vi "RCV Test_ks5080A.vi"(0 "Semiconductor Module Context":T2, 1 "Meas Type":T6, 2 "Test Information":T5={"Exp Name"="Cold Switching", "Lot"="0233A", "Wafer"="15", "Die Type"="L22", "Die X "="6", "Die Y"="8", "Exp"="1", "Die X_Y"="8"}, 3 "# of Cycles":string, 5 "Sweep Settings":T3={"Start"=0.0, "Stop"=1.0, "Step"=0.0}, 7 "Test_Pins":T4={"RF_Pins"=["RF1", "RF2"], "Contact_Meas_Pins"=["RF1"], "Contact_Source_Pins"=["RF1"], "Sweep_Bias_Pins"=[]}, 9 "error in (no error)":errorcluster, 12 "Averaging Count":i32=3, 13 "Plots FilePath":path=path "C:/Users/DalLab/Desktop/Test Data/Plots") -> (4 "ks5080A_Meaurements":T7, 15 "error out":errorcluster)   [LabVIEW 2013]
doc: "Initiates and fetches niVNA S11 measurements and converts it to a capacitance measurement."
uses:
  <vilib>/NI_TestStand_SemiconductorModule/NI_TestStand_Semiconductor_Module.lvlibp/PinMap/General/SemiconductorModuleContext.ctl
  Controls/Sweep Settings.ctl
  Controls/Test_Pins.ctl
  Controls/Test Information.ctl
  Controls/Meas Type.ctl
  Controls/ks5080A_Measurements.ctl
  <vilib>/NI_TestStand_SemiconductorModule/NI_TestStand_Semiconductor_Module.lvlibp
panel:
  in  "Tab Control":enum32{"Graphs", "Controls and Indicators"}(tab)
  out "Graph Cluster":T1
  out "Wafer":string
  out "Die Type":string
  out "Measurement":string
  out "Die X_Y":string
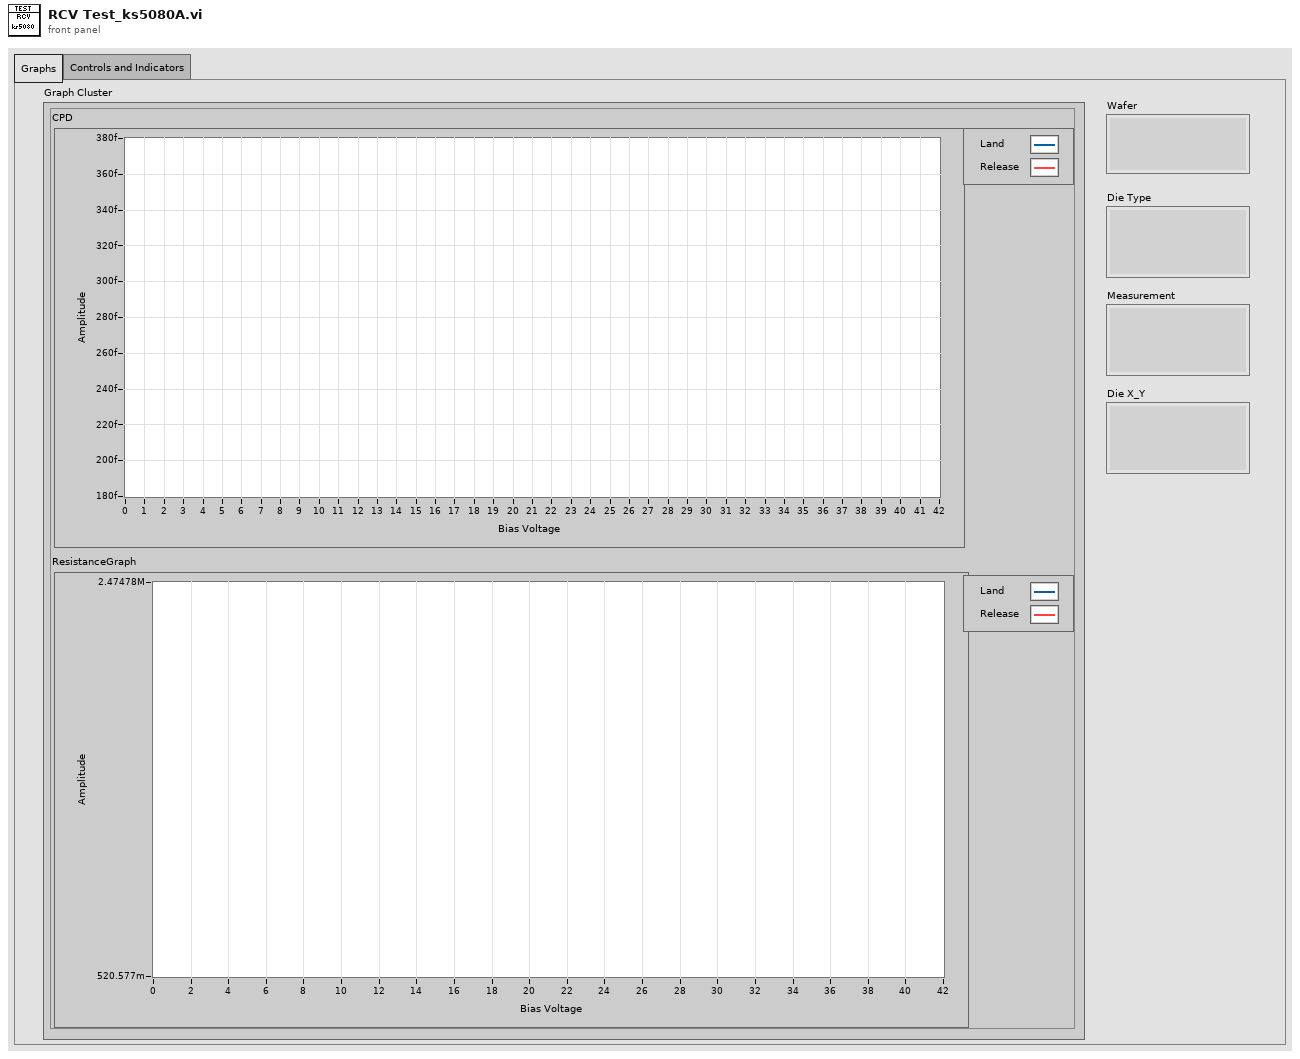
[diagram p1: front panel]
types:
  T1 = cluster{"ResistanceGraph":cluster{dbl[], dbl[]}[], "CPD":cluster{dbl[], dbl[]}[]}
  T2 = typedef "NI_TestStand_Semiconductor_Module.lvlibp/SemiconductorModuleContext.ctl" = refnum<k7>
  T3 = typedef "Sweep Settings.ctl" = cluster{"Start":dbl, "Stop":dbl, "Step":dbl}
  T4 = typedef "Test_Pins.ctl" = cluster{"RF_Pins":string[], "Contact_Meas_Pins":string[], "Contact_Source_Pins":string[], "Sweep_Bias_Pins":string[]}
  T5 = typedef "Test Information.ctl" = cluster{"Exp Name":string, "Lot":string, "Wafer":string, "Die Type":string, "Die X ":string, "Die Y":string, "Exp":string, "Die X_Y":string}
  T6 = typedef "Meas Type.ctl" = enum16{"Floor", "Roof", "Buckling", "Charge Transfer"}
  T7 = typedef "ks5080A_Measurements.ctl" = cluster{"Bias_Sweep_Setting":dbl[], "Bias_voltage measurements":dbl[], "Bias_current measurements":dbl[], "P1_Capacitance":dbl[], "P2_Capacitance":dbl[], "DMM_Measurement_V":dbl[], "Contact_Source Current measurements":dbl[], "Contact_Sink Current measurements":dbl[], "Calculated_Resistance":dbl[], "P3_Capacitance":dbl[], "Port 1_S_parm":string[], "Port 2_S_parm":string[], "Port 3_S_parm":string[]}
  T8 = typedef "ENA_Marker Measurements.ctl" = cluster{"Port 1 Capacitance":dbl[], "Port 2 Capacitance":dbl[], "Port 3 Capacitance":dbl[], "Port 1_S_parm":string[], "Port 2_S_parm":string[], "Port 3_S_parm":string[]}
  T9 = typedef "imagedata.ctl" = cluster{"image type":i32, "image depth":i32, "image":u8[], "mask":u8[], "colors":u32[], "Rectangle":cluster{"left":i16, "top":i16, "right":i16, "bottom":i16}}
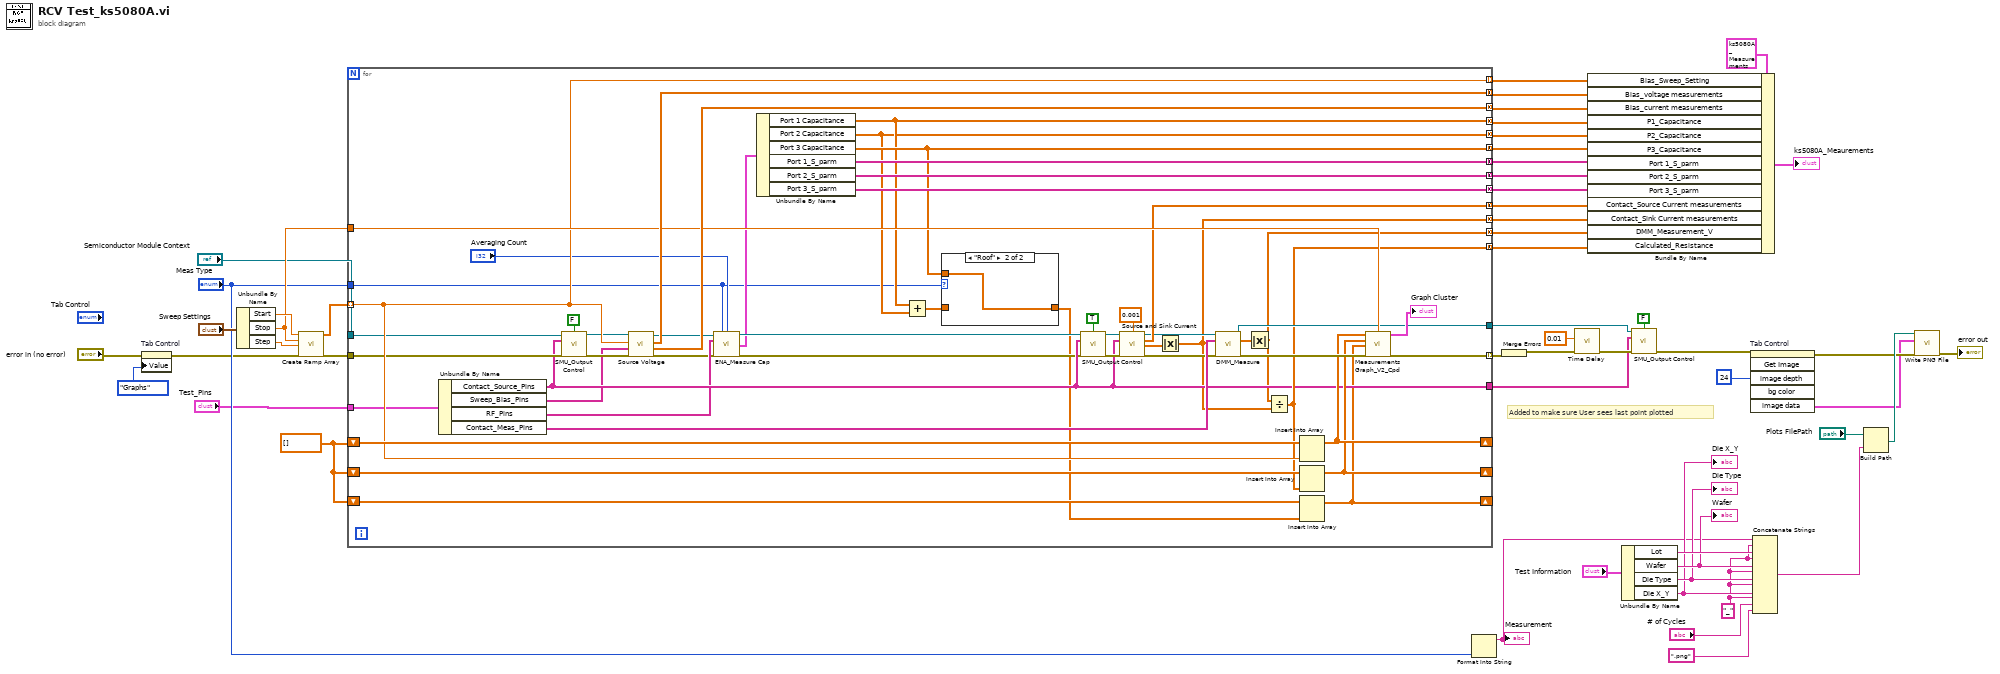
[diagram p0: block diagram]
diagram:
  w6 = "_"
  w46 = dbl[] []
  # "Added to make sure User sees last point plotted"
  n1 = property on="Tab Control" class="TabCtl (strict)"(error in="error in (no error)", "Value"=enum32{"Graphs", "Controls and Indicators"}."Graphs" ("Tab Control")) -> (error out=w7:errorcluster)  [unwired: 1 in, 1 out]
  n2 = Unbundle By Name("Sweep Settings") -> ("Start"=w49:dbl, "Stop"=w47:dbl, "Step"=w48:dbl)
  n3 = call "Create Ramp Array.vi"("Start"=w49, "Stop"=w47, "Step"=w48, "Error In"=w7) -> ("Ramp Pattern"=w52:dbl[], "Error Out"=w2:errorcluster)  [unwired: 10 in]
  n4 = for {
    tunnel: w52 -> [w91] mode=indexing
    tunnel: [w103] -> w38 mode=concatenating
    tunnel: [w102] -> w37 mode=concatenating
    tunnel: [w60] -> w34 mode=concatenating
    tunnel: [w100] -> w51 mode=indexing
    tunnel: w2 -> [w90]
    tunnel: w47 -> [w97]
    shift-right: [w96] -> _
    shift-left: w46 -> [w95]
    shift-right: [w94] -> _
    shift-left: w46 -> [w93]
    shift-right: [w76] -> _
    shift-left: w46 -> [w92]
    tunnel: [w91] -> w39 mode=indexing
    tunnel: [w84] -> w41
    tunnel: [w77] -> w40
    tunnel: [w83] -> w36 mode=concatenating
    tunnel: [w57] -> w35 mode=concatenating
    tunnel: [w82] -> w33 mode=concatenating
    tunnel: [w62] -> w21 mode=concatenating
    tunnel: [w61] -> w20 mode=concatenating
    tunnel: [w63] -> w19 mode=concatenating
    tunnel: [w66] -> w18 mode=concatenating
    tunnel: [w65] -> w17 mode=concatenating
    tunnel: [w64] -> w16 mode=concatenating
    tunnel: "Meas Type" -> [w56]
    tunnel: "Semiconductor Module Context" -> [w54]
    tunnel: "Test_Pins" -> [w53]
    n5 = Unbundle By Name(w53) -> ("Contact_Source_Pins"=w77:string[], "Sweep_Bias_Pins"=w75:string[], "RF_Pins"=w73:string[], "Contact_Meas_Pins"=w98:string[])
    n6 = call "SMU_Output Control.vi"("Semiconductor Module Context"=w54, "output enabled?"=FALSE, "Pins"=w77, "error in (no error)"=w90) -> ("Semiconductor Module Context Out"=w88:T2, "error out"=w89:errorcluster)  [unwired: 10 in]
    n7 = call "Source Voltage.vi"("error in (no error)"=w89, "Pins"=w75, "voltage level"=w91, "Semiconductor Module Context"=w88) -> ("error out"=w55:errorcluster, "current measurements"=w102:dbl[], "voltage measurements"=w103:dbl[], "Semiconductor Module Context Out"=w72:T2)  [unwired: 4 in]
    n8 = call "ENA_Measure Cap.vi"("Semiconductor Module Context"=w72, "Meas Type"=w56, "Averaging Count"="Averaging Count", "Pins"=w73, "error in (no error)"=w55) -> ("Semiconductor Module Context Out"=w71:T2, "Marker Measurements"=w67:T8, "error out"=w74:errorcluster)  [unwired: 8 in]
    n9 = Unbundle By Name(w67) -> ("Port 1 Capacitance"=w62:dbl[], "Port 2 Capacitance"=w61:dbl[], "Port 3 Capacitance"=w63:dbl[], "Port 1_S_parm"=w66:string[], "Port 2_S_parm"=w65:string[], "Port 3_S_parm"=w64:string[])
    n10 = Add(x=w62, y=w61) -> (x+y=w70:dbl[])
    n11 = case shown="\"Roof\"" w56 {
      tunnel: w70 -> [w104 _]
      tunnel: [w104 w105] -> w68
      tunnel: w63 -> [_ w105]
      frame "Floor", Default {
      }
      frame "Roof" {
      }
    }
    n12 = call "SMU_Output Control.vi"("Semiconductor Module Context"=w71, "output enabled?"=TRUE, "Pins"=w77, "error in (no error)"=w74) -> ("Semiconductor Module Context Out"=w78:T2, "error out"=w79:errorcluster)  [unwired: 10 in]
    n13 = call "Source and Sink Current.vi"("Semiconductor Module Context"=w78, "Current level"=0.001, "Pins"=w77, "error in (no error)"=w79) -> ("Semiconductor Module Context Out"=w80:T2, "Source Current measurements"=w83:dbl[], "Sink Current measurements"=w58:dbl[], "error out"=w81:errorcluster)  [unwired: 8 in]
    n14 = Absolute Value(x=w58) -> (abs(x)=w57:dbl[])
    n15 = call "DMM_Measure.vi"("Semiconductor Module Context"=w80, "Pins"=w98, "Error In"=w81) -> ("Semiconductor Module Context Out"=w84:T2, "Measurement"=w59:dbl[], "Error Out"=w101:errorcluster)  [unwired: 10 in]
    n16 = Absolute Value(x=w59) -> (abs(x)=w60:dbl[])
    n17 = Divide(x=w60, y=w57) -> (x/y=w82:dbl[])
    n18 = Insert Into Array(array=w95, new element=w91) -> (w96:dbl[])  [unwired: 1 in]
    n19 = Insert Into Array(array=w93, new element=w82) -> (w94:dbl[])  [unwired: 1 in]
    n20 = Insert Into Array(array=w92, new element=w68) -> (w76:dbl[])  [unwired: 1 in]
    n21 = call "Measurements Graph_V2_Cpd.vi"("Bias Voltage"=w96, "Stop_V"=w97, "Resitance"=w94, "Cpd"=w76, "Error In"=w101) -> ("Graph Cluster"=→"Graph Cluster":T1, "Error Out"=w100:errorcluster)  [unwired: 9 in]
  }
  n22 = Format Into String("Meas Type") -> (resulting string=w15:string)  [unwired: 3 in, 1 out]
  "Measurement" <- w15
  n23 = Merge Errors(w51) -> (w44:errorcluster)
  n24 = call "Time Delay"("error in (no error)"=w44, "Delay Time (s)"=0.01) -> ("error out"=w42:errorcluster)  [unwired: 9 in]
  n25 = Bundle By Name(cluster=T7 {"Bias_Sweep_Setting"=[], "Bias_voltage measurements"=[], "Bias_current measurements"=[], "P1_Capacitance"=[], "P2_Capacitance"=[], "DMM_Measurement_V"=[], "Contact_Source Current measurements"=[], "Contact_Sink Current measurements"=[], "Calculated_Resistance"=[], "P3_Capacitance"=[], "Port 1_S_parm"=[], "Port 2_S_parm"=[], "Port 3_S_parm"=[]} ("ks5080A_Meaurements 2"), "Bias_Sweep_Setting"=w39, "Bias_voltage measurements"=w38, "Bias_current measurements"=w37, "P1_Capacitance"=w21, "P2_Capacitance"=w20, "P3_Capacitance"=w19, "Port 1_S_parm"=w18, "Port 2_S_parm"=w17, "Port 3_S_parm"=w16, "Contact_Source Current measurements"=w36, "Contact_Sink Current measurements"=w35, "DMM_Measurement_V"=w34, "Calculated_Resistance"=w33) -> (→"ks5080A_Meaurements":T7)
  n26 = Unbundle By Name("Test Information") -> ("Lot"=w31:string, "Wafer"=w30:string, "Die Type"=w29:string, "Die X_Y"=w28:string)
  "Wafer" <- w30
  "Die Type" <- w29
  "Die X_Y" <- w28
  n27 = call "SMU_Output Control.vi"("Semiconductor Module Context"=w41, "output enabled?"=FALSE, "Pins"=w40, "error in (no error)"=w42) -> ("error out"=w13:errorcluster)  [unwired: 10 in, 1 out]
  n28 = invoke on="Tab Control" class="TabCtl (strict)" method="Get Image"(error in=w13, "image depth"=24 ("Image Depth")) -> (error out=w12:errorcluster, "image data"=w11:T9)  [unwired: 4 in, 4 out]
  n29 = Concatenate Strings(w15, w6, w31, w6, w30, w6, w29, w6, w28, w6, "# of Cycles", ".png" ("string")) -> (w27:string)
  n30 = Build Path(base path="Plots FilePath", name or relative path=w27) -> (appended path=w25:path)
  n31 = call <vilib>:"Write PNG File.vi"("error in (no error)"=w12, "image data"=w11, "path to PNG file"=w25) -> ("error out"=→"error out":errorcluster)  [unwired: 7 in, 1 out]
